vi "Iterate Grid.vi"(10 "Iteration Attempts":u16, 11 "Grid.lvclass 2":refnum<class "Grid.lvclass">) -> (3 "Grid.lvclass":refnum<class "Grid.lvclass">)   [LabVIEW 2016, in "Pixel.lvclass"]
uses:
  Classes/Pixel/Pixel.lvclass
  Classes/Grid/Grid.lvclass
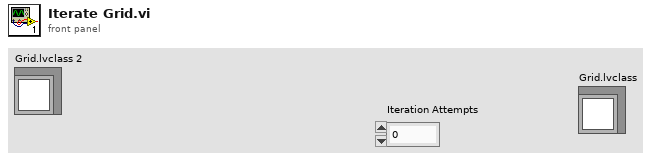
[diagram p1: front panel]
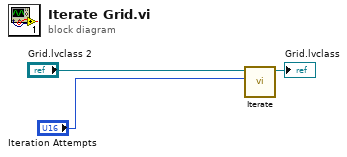
[diagram p0: block diagram]
diagram:
  n1 = call "Iterate.vi"("Iterations"="Iteration Attempts", "Grid.lvclass 2"="Grid.lvclass 2") -> ("Grid.lvclass"=→"Grid.lvclass":refnum<class "Grid.lvclass">)  [unwired: 9 in]
